vi "test_leduri.vi"() -> ()   [LabVIEW 2009]
uses:
  <vilib>/Platform/portaccess.llb/Out Port8.vi
panel:
  out "Boolean 2":bool
  in  "stop":bool
  in  "Start":bool
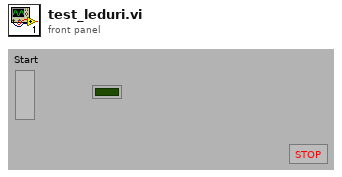
[diagram p1: front panel]
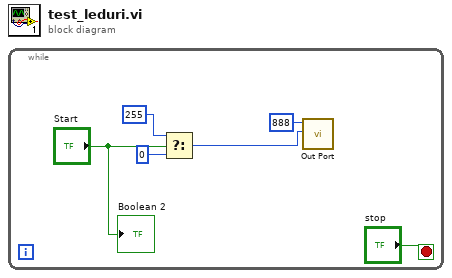
[diagram p0: block diagram]
diagram:
  n1 = while {
    stop <- "stop" stop-if-true
    n2 = Select(t=u8 255 ("write value"), s="Start", f=u8 0) -> (s? t:f=w3:u8)
    n3 = call-poly <vilib>:"Out Port.vi"("write value"=w3, "address"=i16 888) -> ()  [unwired: 7 in, 1 out]
    "Boolean 2" <- "Start"
  }
